vi "update_action_combobox.vi"() -> ()   [LabVIEW 2018]
panel:
  in  "Write To Action Control":bool
  in  "Action":string(combo)
  in  "Values":string[](array[string])
  in  "Strings":string[](array[string])
  # "a\nb\nc\nd\ne\nf\ng\nh\ni\nj\nk\nl\nm\nn\no\np\nq\nr\ns\nt\nu\nv\nw\nx\ny\nz"
  # "1\n2\n3\n4\n5\n6\n7\n8\n9\n10\n11\n12\n13\n14\n15\n16\n17\n18\n19\n20\n21\n22\n23\n24\n25\n26"
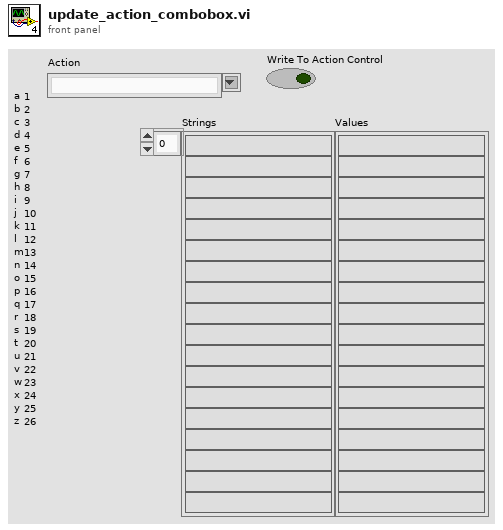
[diagram p1: front panel]
types:
  T1 = typedef "LVComboBoxStrsAndValuesArrayTypeDef.ctl" = cluster{"String":string, "Value":string}[]
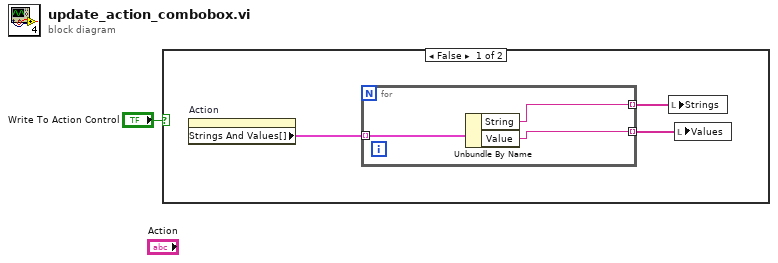
[diagram p0: block diagram]
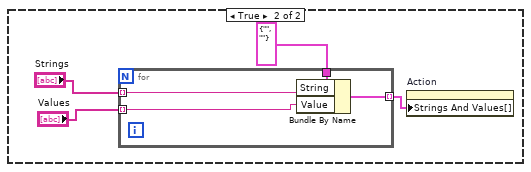
[diagram p2: hidden frame]
diagram:
  n1 = case shown="False" "Write To Action Control" {
    frame False {
      n2 = property on="Action" class="CmbBox"() -> ("Strings And Values[]"=w4:T1)  [unwired: 2 in, 2 out]
      n3 = for {
        tunnel: w4 -> [w7] mode=indexing
        tunnel: [w6] -> w3 mode=indexing
        tunnel: [w5] -> w2 mode=indexing
        n4 = Unbundle By Name(w7) -> ("String"=w6:string, "Value"=w5:string)
      }
      n5 = local write "Strings"(w3) -> ()
      n6 = local write "Values"(w2) -> ()
    }
    frame True {
      n7 = for {
        tunnel: cluster{"String":string, "Value":string} {"String"="", "Value"=""} -> [w15]
        tunnel: "Strings" -> [w14] mode=indexing
        tunnel: "Values" -> [w13] mode=indexing
        tunnel: [w12] -> w8 mode=indexing
        n8 = Bundle By Name(cluster=w15, "String"=w14, "Value"=w13) -> (w12:cluster{"String":string, "Value":string})
      }
      n9 = property on="Action" class="CmbBox"("Strings And Values[]"=w8) -> ()  [unwired: 2 in, 2 out]
    }
  }
